vi "Devices by Direction.vi"(8 "error in (no error)":errorcluster, 10 "Direction":T1, 11 "VoiceMeeterRemote in":refnum<class "VoiceMeeterRemote.lvclass">) -> (0 "error out":errorcluster, 2 "Device Count":i32, 3 "VoiceMeeterRemote out":refnum<class "VoiceMeeterRemote.lvclass">)   [LabVIEW 2022 SP3, in "VoiceMeeterRemote.lvlib" / "VoiceMeeterRemote.lvclass"]
doc: "Returns the number of devices for the specified input / output direction. This will depend on the type of Voicemeeter application that is connected to.\n\nVoicemeeter has 3 devices.\nBanana has 5 devices.\nPotato has 8 devices."
uses:
  VoiceMeeterRemote.lvclass
  Direction.ctl
  VoiceMeeterRemote.lvclass/VoiceMeeterRemote.ctl
  VoiceMeeterRemote.lvlib
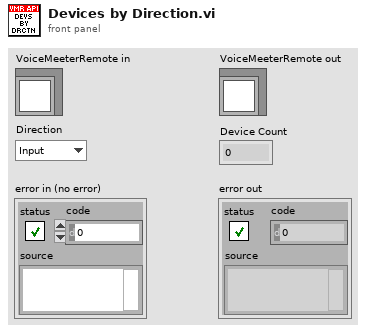
[diagram p1: front panel]
types:
  T1 = typedef "VoiceMeeterRemote.lvlib/Direction.ctl" = enum16{"Input", "Output"}
  T2 = typedef "VoiceMeeterRemote.lvlib/Voicemeeter Type.ctl" = enum16{"Unknown", "Voicemeeter", "Banana", "Potato", "Potato x64"}
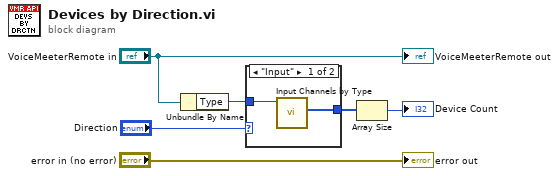
[diagram p0: block diagram]
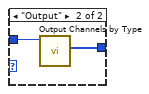
[diagram p2: hidden frame]
diagram:
  n1 = Unbundle By Name("VoiceMeeterRemote in") -> ("Type"=w3:T2)
  n2 = case shown="\"Input\"" "Direction" {
    tunnel: w3 -> [w8 w10]
    tunnel: [w7 w9] -> w2
    frame "Input" {
      n3 = call "Input Channels by Type.vi"("Voicemeeter Type"=w8) -> ("Channel Count"=w7:i32[])  [unwired: 10 in]
    }
    frame "Output" {
      n4 = call "Output Channels by Type.vi"("Voicemeeter Type"=w10) -> ("Channel Count"=w9:i32[])  [unwired: 10 in]
    }
  }
  n5 = Array Size(array=w2) -> (size(s)=→"Device Count":i32)
  "error out" <- "error in (no error)"
  "VoiceMeeterRemote out" <- "VoiceMeeterRemote in"
